vi "Single_channel_data_change.vi"(10 "String":string, 11 "element in":waveform(dbl)) -> (2 "element out":waveform(dbl))   [LabVIEW 2024]
panel:
  in  "Array - String":string[](array[string])
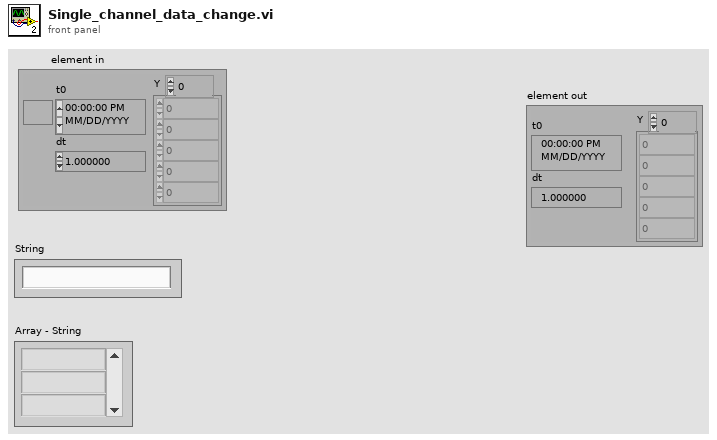
[diagram p1: front panel]
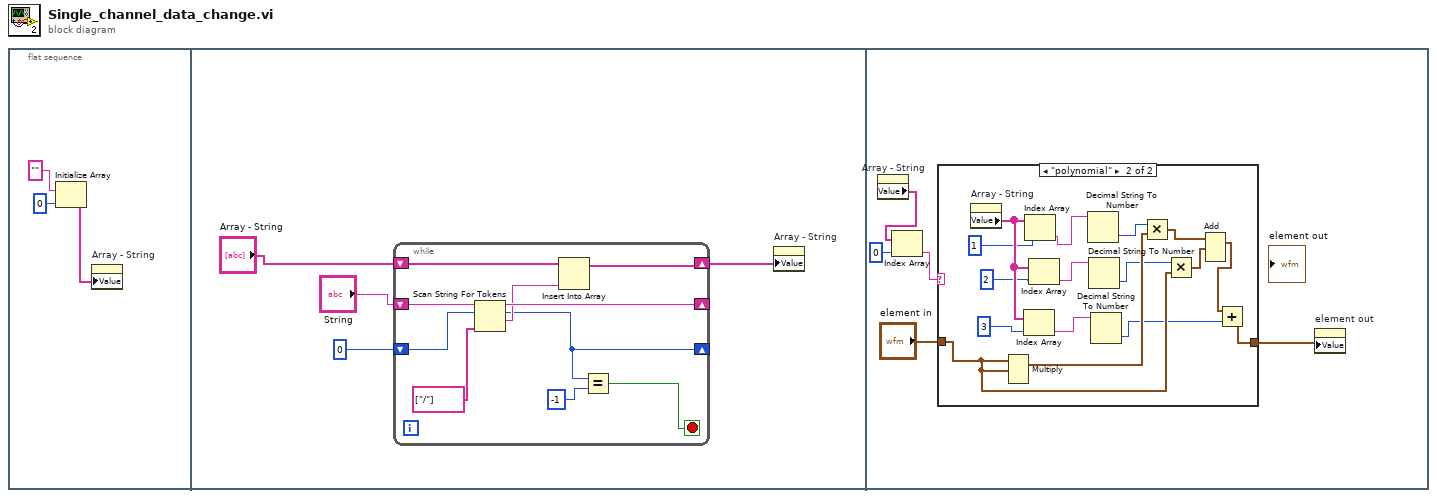
[diagram p0: block diagram]
diagram:
  n1 = flat-sequence {
    frame #0 {
      n2 = Initialize Array("", 0 ("dimension size")) -> (w1:string[])
      n3 = property on="Array - String" class="Arr (strict)"("Value"=w1) -> ()  [unwired: 2 in, 2 out]
    }
    frame #1 {
      n4 = while {
        shift-right: [w16] -> _
        shift-left: "String" -> [w17]
        shift-right: [w11] -> w4
        shift-left: "Array - String" -> [w13]
        shift-right: [w10] -> _
        shift-left: 0 -> [w15]
        stop <- w8 stop-if-true
        n5 = Scan String For Tokens(6:string[] ["/"] ("delimiters (\\s,\\t,\\r,\\n)"), 8:w15, 9:w17) -> (1:w12:string, 2:w10:i32, 3:w16:string)  [unwired: 3 in, 1 out]
        n6 = Insert Into Array(array=w13, new element=w12) -> (w11:string[])  [unwired: 1 in]
        n7 = Equal?(x=w10, y=-1) -> (x = y?=w8:bool)
      }
      n8 = property on="Array - String" class="Arr (strict)"("Value"=w4) -> ()  [unwired: 2 in, 2 out]
    }
    frame #2 {
      n9 = property on="Array - String" class="Arr (strict)"() -> ("Value"=w22:string[])  [unwired: 2 in, 2 out]
      n10 = Index Array(array=w22, index=0) -> (element=w20:string)
      n11 = case shown="\"polynomial\"" w20 {
        tunnel: "element in" -> [w23 w31]
        tunnel: [w23 w27] -> w18
        frame "original", Default {
        }
        frame "polynomial" {
          n12 = property on="Array - String" class="Arr (strict)"() -> ("Value"=w39:string[])  [unwired: 2 in, 2 out]
          n13 = Multiply(1:w31, 2:w31) -> (0:w32:waveform(dbl))  [unwired: 1 in, 1 out]
          n14 = Index Array(array=w39, index=3) -> (element=w33:string)
          n15 = Index Array(array=w39, index=1) -> (element=w35:string)
          n16 = Index Array(array=w39, index=2) -> (element=w34:string)
          n17 = Decimal String To Number(string=w35) -> (number=w25:i32)  [unwired: 2 in, 1 out]
          n18 = Decimal String To Number(string=w34) -> (number=w26:i32)  [unwired: 2 in, 1 out]
          n19 = Decimal String To Number(string=w33) -> (number=w24:i32)  [unwired: 2 in, 1 out]
          n20 = Multiply(x=w25, y=w32) -> (x*y=w30:waveform(dbl))
          n21 = Multiply(x=w26, y=w31) -> (x*y=w29:waveform(dbl))
          n22 = Add(1:w29, 2:w30) -> (0:w28:waveform(dbl))  [unwired: 1 in, 1 out]
          n23 = Add(x=w28, y=w24) -> (x+y=w27:waveform(dbl))
        }
      }
      n24 = property on="element out" class="WFD (strict)"("Value"=w18) -> ()  [unwired: 2 in, 2 out]
    }
  }
